vi "Run CSM Module.vi"(7 "CSM-Module":string, 8 "Error in":errorcluster caption="Error in (no error)", 11 "CSM-Instance":string) -> (0 "Error out":errorcluster)   [LabVIEW 2020, in "CSM-ModuleManager.lvlib"]
uses:
  CSM-ModuleManager.lvlib
  Operation.ctl
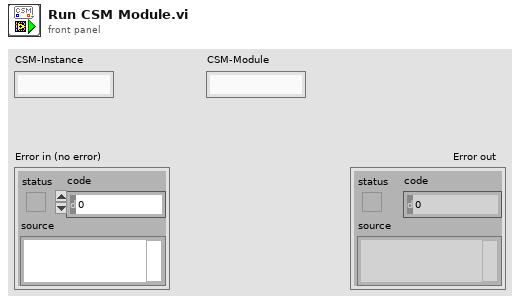
[diagram p1: front panel]
types:
  T1 = typedef "CSM-ModuleManager.lvlib/Operation.ctl" = enum16{"Register", "UnRegister", "Load Config", "Get"}
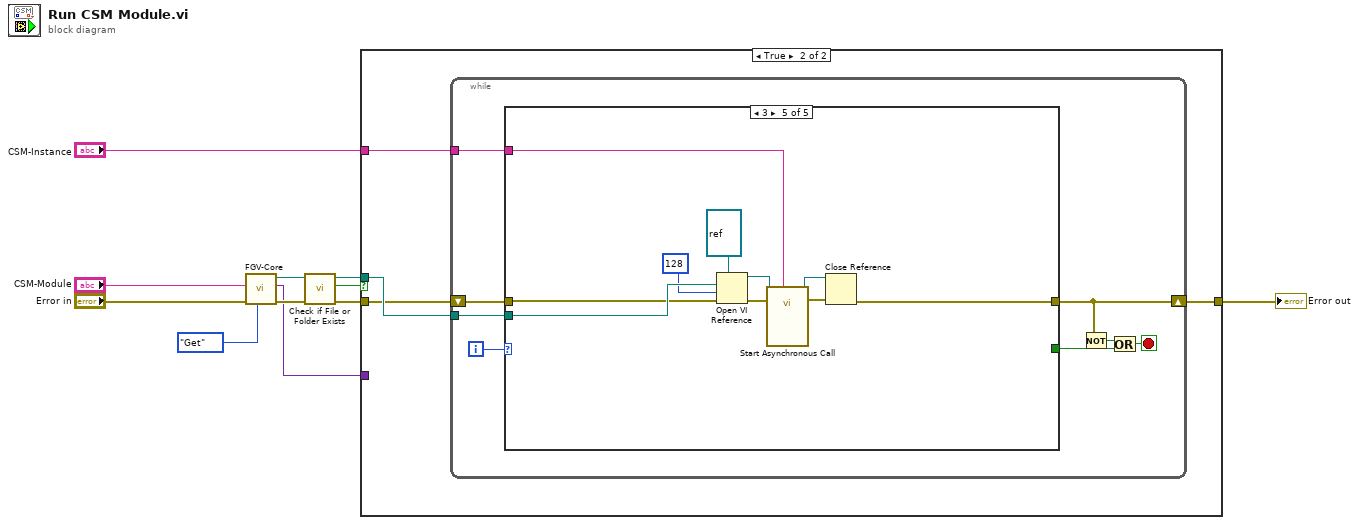
[diagram p0: block diagram]
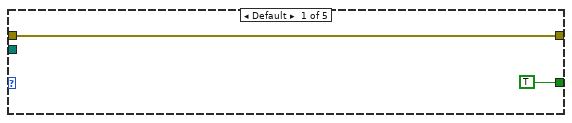
[diagram p3: hidden frame]
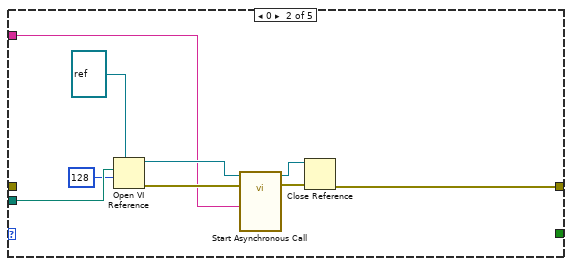
[diagram p4: hidden frame]
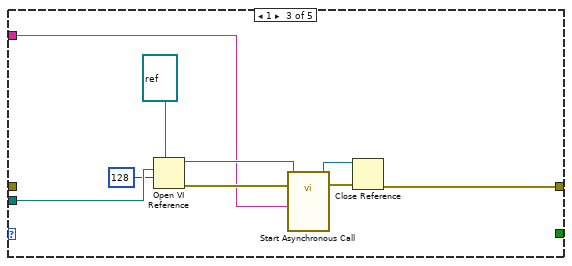
[diagram p5: hidden frame]
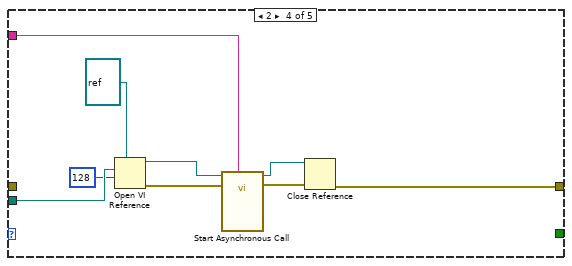
[diagram p6: hidden frame]
diagram:
  n1 = call "FGV-Core.vi"("Enum"=Operation."Get", "error in (no error)"="Error in", "csm"="CSM-Module") -> ("error out"=w4:errorcluster, "Variant"=w1:variant, "Path"=w7:path)  [unwired: 6 in]
  n2 = call <vilib>:"Check if File or Folder Exists.vi"("error in (no error)"=w4, "path"=w7) -> ("error out"=w3:errorcluster, "file or folder exists?"=w2:bool, "dup path"=w5:path)  [unwired: 7 in]
  n3 = case shown="True" w2 {
    tunnel: [w12 w16] -> w8
    tunnel: "CSM-Instance" -> [_ w15]
    tunnel: w5 -> [_ w14]
    tunnel: w3 -> [w12 w13]
    tunnel: w1 -> [_ _]
    frame False {
    }
    frame True {
      n4 = while {
        tunnel: w14 -> [w24]
        shift-right: [w19] -> w16
        shift-left: w13 -> [w21]
        tunnel: w15 -> [w17]
        i -> [w23]
        stop <- w20 stop-if-true
        n5 = case shown="3" w23 {
          tunnel: w24 -> [_ w33 w42 w51 w60]
          tunnel: [w25 w32 w41 w50 w59] -> w19
          tunnel: [TRUE _ _ _ _] -> w22
          tunnel: w21 -> [w25 _ _ _ w54]
          tunnel: w17 -> [_ w28 w37 w46 w56]
          frame Default {
          }
          frame 0 {
            n6 = Open VI Reference(type specifier VI Refnum (for type only)=refnum<vi> refnum, vi path=w33, options=128) -> (vi reference=w35:refnum<vi>, error out=w34:errorcluster)  [unwired: 3 in]
            n7 = call-by-ref "Start Asynchronous Call"(reference=w35, error in=w34, "Init State(\"Macro: Initialize\")"=w28) -> (reference out=w30:refnum<vi>, error out=w29:errorcluster)  [unwired: 11 in]
            n8 = Close Reference(reference=w30, error in (no error)=w29) -> (error out=w32:errorcluster)
          }
          frame 1 {
            n9 = Open VI Reference(type specifier VI Refnum (for type only)=refnum<vi> refnum, vi path=w42, options=128) -> (vi reference=w44:refnum<vi>, error out=w43:errorcluster)  [unwired: 3 in]
            n10 = call-by-ref "Start Asynchronous Call"(reference=w44, error in=w43, "Current Module(\"\" to generate an ID)"=w37) -> (reference out=w39:refnum<vi>, error out=w38:errorcluster)  [unwired: 11 in]
            n11 = Close Reference(reference=w39, error in (no error)=w38) -> (error out=w41:errorcluster)
          }
          frame 2 {
            n12 = Open VI Reference(type specifier VI Refnum (for type only)=refnum<vi> refnum, vi path=w51, options=128) -> (vi reference=w53:refnum<vi>, error out=w52:errorcluster)  [unwired: 3 in]
            n13 = call-by-ref "Start Asynchronous Call"(reference=w53, error in=w52, "Current Module(\"\" to generate an ID)"=w46) -> (reference out=w47:refnum<vi>, error out=w48:errorcluster)  [unwired: 11 in]
            n14 = Close Reference(reference=w47, error in (no error)=w48) -> (error out=w50:errorcluster)
          }
          frame 3 {
            n15 = Open VI Reference(type specifier VI Refnum (for type only)=refnum<vi> refnum, vi path=w60, options=128, error in (no error)=w54) -> (vi reference=w62:refnum<vi>, error out=w61:errorcluster)  [unwired: 2 in]
            n16 = call-by-ref "Start Asynchronous Call"(reference=w62, error in=w61, "Current Module(\"\" to generate an ID)"=w56) -> (reference out=w57:refnum<vi>, error out=w63:errorcluster)  [unwired: 11 in]
            n17 = Close Reference(reference=w57, error in (no error)=w63) -> (error out=w59:errorcluster)
          }
        }
        n18 = Not(x=w19) -> (.not. x?=w18:bool)
        n19 = Or(x=w18, y=w22) -> (x .or. y?=w20:bool)
      }
    }
  }
  "Error out" <- w8
